vi "AlliGator Display Accumulated Dataset.vi"(8 "error in (no error)":errorcluster, 9 "Sum (F) or Average (T)":bool, 11 "AlliGator IV DVR in":refnum<data-value>) -> (0 "error out":errorcluster, 1 "Averaged?":bool, 2 "# Accumulated Datasets":i32, 3 "AlliGator IV DVR out":refnum<data-value>, 7 "Time-Series Folder":path)   [LabVIEW 2021, in "AlliGator Source Image.lvlib"]
doc: "Displays the Sum of all accumulated images or their mean, depending on the user-selected menu option."
uses:
  AlliGator Source Image.lvlib
  AlliGator Internal Variables v2.ctl
  <vilib>/vision/Image Controls.llb/IMAQ Image.ctl
  AlliGator Gate Image Set.ctl
  AlliGator FLI Dataset Type.ctl
  AlliGator Data Series Type.ctl
  AlliGator Dataset Channel.ctl
  AlliGator Gate Arithmetic.ctl
  AlliGator Displayed Image.ctl
  Image/Named ROI Description.ctl
  AlliGator Decay Metadata v3.ctl
  AlliGator Decay Background Subtraction Info.ctl
  AlliGator Baseline Subtraction Method.ctl
  Graphs/XY Graph/XY Graph Plot Shift Parameters.ctl
  Graphs/XY Graph/XY Graph Plot Shift Method.ctl
  AlliGator Decay Extrapolation Parameters.ctl
  Phasor/Calibration Phasor (m, phi).ctl
  Phasor/Phasor Reference Series.ctl
  Phasor/Phasor Calibration Map v2.ctl
  Phasor/Phasor (g, s).ctl
  AlliGator Raw Phasor Plot Data v4.ctl
  Phasor/Phasor Standard Deviation Options.ctl
  AlliGator Phasor Multi-Harmonic Data.ctl
  Phasor/Phasor Harmonic Data.ctl
  AlliGator Decay Fit Options & Parameters v2.ctl
  Fits/IRF(X)PSED/Decay Fit Options v2.ctl
  Fits/Decay Convolution/Decay Model.ctl
  Fits/Residual Type.ctl
  Fits/IRF(X)PSED/Fit Weights Type.ctl
  Fits/Non-linear Fitting Method v2.ctl
  Fits/Fit Calculation Method.ctl
  Fits/Non-linear Fitting Algorithm.ctl
  AlliGator Decay Fit Parameter Constraints 2.ctl
  Fits/IRF(X)PSED/Decay Fit Parameters In List.ctl
  Fits/IRF(X)PSED/MLE Baseline Offset Type.ctl
  AlliGator Decay Preprocessing Parameters.ctl
  Fits/IRF(X)PSED/Decay Fit Parameters & Derived Quantities List.ctl
  AlliGator Parameter Maps Data.ctl
  AlliGator Variables List.ctl
  Variant/Variant to Data/Variant to I32.vi
  Variant/Variant to Data/Variant to U16.vi
  <vilib>/vision/NI_Vision_Development_Module.lvlib
  Variant/Variant to Data/Variant to Data.lvlib
  AlliGator Globals, Variables & Constants.lvlib
  Utilities/Utilities.lvlib
  Phasor/Phasor.lvlib
  Image/Image.lvlib
  AlliGator Internal Variables.lvlib
  AlliGator Files.lvlib
  AlliGator Phasor Graph.lvlib
  AlliGator Decay Preprocessing.lvlib
  Graphs/XY Graph/XY Graph Add-Ons.lvlib
  AlliGator Phasor Plot.lvlib
  Fits/Fits.lvlib
  AlliGator Decay Fit.lvlib
  AlliGator Decay Fit Parameter Map.lvlib
  AlliGator Settings.lvlib
  AlliGator Dual-Channel Datasets.lvlib
panel:
  # "see the AlliGator License on the block diagram (Ctrl+E or Window:Show Block Diagram)"
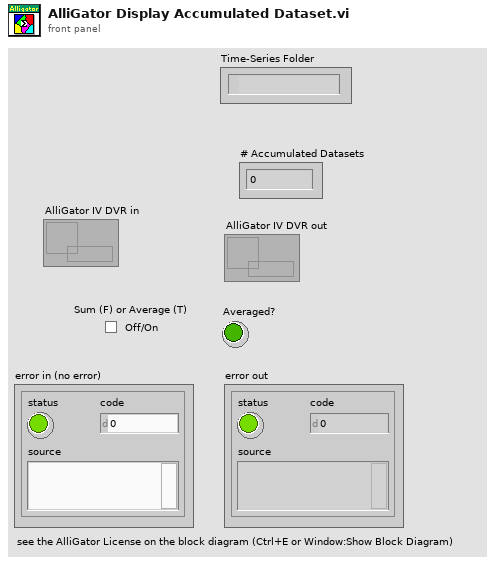
[diagram p1: front panel]
types:
  T1 = typedef "AlliGator Globals, Variables & Constants.lvlib/AlliGator Variables List.ctl" = enum16{"---- GUI ----", "GUI:Initialization Status", "GUI:State Indicators Refnum", "GUI:Original AlliGator Menu Items", "GUI:Current Action Loop State", "GUI:Script in progress", "GUI:Playback", "GUI:Loop Playback", "GUI:Search ROI Used", "GUI:Search ROI", "Decay Graph Max Legend Size", "Intensity Graph Max Legend Size", "Decay Statistics Graph Max Legend Size", "Phasor Graph Max Legend Size", "Phasor Ratio Graph Max Legend Size", "Lifetime Graph Max Legend Size", "---- Files ----", "Files:Export Dataset Frames as Individual Files", "Files:Show Batch Export Help Balloons", "Files:Frames in Dataset", "Files:ptu File Frame Start Indices", "Files:Current Frame in Dataset", "Files:Current Frame Timestamp", "Files:Dataset Loaded", "Files:Dataset Metadata", "Files:Dataset Channel", "Files:Dataset Data Description", "Files:Background Dataset Metadata", "Files:Background Dataset Channel", "Files:Background Dataset Data Description", "Files:Background File Subtraction", "Files:Background File Path", "Files:Background File Pile-up Correction", "Files:Background File Pixel Well Capacity", "Files:Background File Scaling Factor", "Files:Current Dataset Load Settings", "Files:Dataset Path", "------ Python Plugins ------", "Python Plugins:Information", "Python Plugins:Python Session", "Python Plugins:Valid Python Session?", "---- Source Image ----", "Source Image:ROIs", "Source Image:Current ROI", "Source Image:ROI Event Refnum", "X_Source Image Display Range", "X_Source Image Palette Information", "Source Image:Palette List", "Source Image:Scale", "Source Image:ROI Overlay Color", "Source Image:ICCD-specific Information", "Source Image:Overlay to Erase", "Source Image:Is Displayed Image Accumulated", "---- Image Profile Window ----", "Image Profile:Overlay ROI in Source Image", "Image Profile Window Event Refnum", "Image Profile:IntensityType", "Image Profile:Intensity Average Type", "Image Profile:Intensity-weighted SDV", "Image Profile:Box Profile Type", "Image Profile Window Open", "Image Profile:Plotted Fit Parameter", "X_Type of Displayed Image", "X_Time Gate Slider", "White Light Image Modified", "Mask Image Modified", "Macrotime Gate Separation", "------ Phasor Graph -------", "Phasor Graph:Show Line", "---- Phasor Plot ---", "Phasor Plot Parameters Changed", "FLI Dataset Modified since last Phasor Plot Calculation", "Phasor Harmonics Data", "Selected Phasor Harmonics", "Phasor Harmonic Manager Event Refnum", "Phasor Plot ROIs", "Current Phasor Plot ROI", "Phasor Plot ROI Event Refnum", "Phasor Plot Image Reference Points", "Phasor Plot Computed", "Phasor Plot Palette Information", "Phasor Plot Palette List", "Phasor Ratio Palette Information", "Phasor Ratio Palette List", "Phasor Image Scale", "Phasor Plot Image Overlay to Erase", "Phasor Plot Image Elements to Update", "Current Phasor Plot Calculation Parameters", "Current Phasor Calibration Options", "Reset Cumulated Phasor Plot", "Phasor Ratio Reference 1", "Phasor Ratio Lifetime Reference 1", "Phasor Ratio Reference 1 Frequency", "Phasor Ratio Reference 2", "Phasor Ratio Lifetime Reference 2", "Phasor Ratio Reference 2 Frequency", "---- Decay Analysis ----", "Number of Selected Decays to Fit", "LS Fit Results", "LAR Fit Results", "BS Fit Results", "Last Decay Max - Min", "Best Fit Parameters", "Best Fit Parameter Names", "Actual Size X", "Actual Size Y", "Binning X", "Binning Y", "Actual # Gates", "Dataset Number", "Gates to...", "Gates Skipped", "Gates to keep", "Gate Step", "Gate Separation", "Reversed Gates", "Pile-up Correction", "Pixel Well Capacity", "Background Subtracted", "Background Subtraction Method", "Background Definition Range", "Background File (deprecated)", "Number of Dataset Accumulated", "Array of Accumulated Dataset Paths", "Do Averaged Datasets", "Destination File Path", "Process Plot Target", "Use 1/D as Phasor Frequency", "---- Decay Fit Parameter Map -----", "Decay Fit Parameter Map Palette Information", "Decay Fit Parameter Map Palette List", "Local Decay Graph Window Event Refnum", "------- Local Decay Window ---------", "Use normalized IRF for convolution", "----- Miscellaneous ----", "Skippable Dialog Windows Status"}
  T2 = typedef "AlliGator Internal Variables.lvlib/AlliGator Internal Variables v2.ctl" = cluster{"Displayed Image":T3, "White Light Image":T3, "Mask Image":T3, "ROI Mask Image":T3, "Current Dataset Images 1":T4, "Background Dataset Images 1":T4, "Current Dataset Images 2":T4, "Background Dataset Images 2":T4, "Current Dataset Arithmetic Images":T4, "Accumulated Dataset Images 1":T4, "Accumulated Dataset Images 2":T4, "Accumulated Dataset Arithmetic Images":T4, "Phasor Plot Image":T3, "Decay Fit Parameter Map Image":T3, "Single Data Point Path":path, "White Light Image Path":path, "Mask Image Path":path, "Time-Series Folder":path, "[Time-Series Paths]":path[], "Current Dataset":i32, "Single Dataset Type":T5, "Current Folder":string, "AlliGator Data Series Type":T6, "# Datasets":i32, "Dual-Channel Dataset":bool, "Selected Channel Name":string, "Dataset Channel":T7, "Channel Arithmetic":T8, "Dual-Channel Background Dataset":bool, "Background Channel":T7, "Dual-Channel Accumulated Dataset":bool, "Start Time":dbl, "[Time-Series Timestamps]":dbl[], "[Intensity Corrections]":dbl[], "Time Series Script":bool, "Type of Displayed Image":T9, "Gate Image Slide":u16, "# Gates":i32, "ROIs":T10[], "ROI Decay":cluster{"t Array":dbl[], "I Array":dbl[]}, "Valid Decay":bool, "Decay  Metadata":T12, "Reference Decay Plot Name":string, "Reference Decay":cluster{"t Array":dbl[], "I Array":dbl[]}, "Decay Shift Plot":cluster{"Time Stamps":dbl[], "Decay Shifts":dbl[]}, "[Decays Max Values]":sgl[], "[Decays Min Values]":sgl[], "Calibration Phasor":T18, "Calibration Phasor Series":T19, "Phasor Calibration Map":T20, "Calibration Map MD5 Digest":string, "Last Raw Phasor":T21, "Last Calibrated Phasor":T21, "Last Calibrated Phasor SDV":T21, "Phasor Graph:Phasor Plot":cluster{"g Array":dbl[], "s Array":dbl[]}, "Phasor Graph:Phasor SDV Plot":cluster{"g Array":dbl[], "s Array":dbl[]}, "[Phasor Graph:Raw Phasor Plots]":T22[], "Phasor Plot locked to Ref 1":i32, "[Phasor Plot(s) locked to Ref 1]":i32[], "[Phasor Plot(s) locked to Ref 2]":i32[], "[Pixel Phasors]":T21[], "[[Sum Image]]":dbl[][], "[[CSG Phasors]]":csg[][], "[[Valid Pixel?]]":bool[][], "I/m/phi Dataset":cluster{"I/m/phi Dataset?":bool, "Base Frequency":dbl[unit], "Harmonic Orders":u8[]}, "Multi Phasor Plot Data":T24, "Decay Fit Options & Parameters":T26, "Fit Options: Decay Preprocessing Parameters":T37, "Fit Options: Reference Decay":cluster{"t Array":dbl[], "I Array":dbl[]}, "Is Full Image Parameters Map":bool, "Is Single-Pixels Parameters Map":bool, "NLSF Parameters Map X Resolution":i32, "NLSF Parameters Map Y Resolution":i32, "[Single Decay Fit Parameters]":dbl[], "Fit Model":T28, "[[Multiple Decays Fit Parameters]]":dbl[][], "[[Multiple Decays Fit Parameter SDVs]]":dbl[][], "[[IRFs]]":dbl[][], "IRF Array Time Axis":dbl[], "Decay Array Time Axis":dbl[], "[Decay Fit Parameter Names]":T38[], "[[Phasor Ratios]]":dbl[][], "[[Average Lifetimes]]":dbl[][], "Amplitude Weighted Average Lifetime":bool, "[Decay Sum]":dbl[], "Parameter Maps":T39[], "[[User-defined Quantities]]":dbl[][], "User-defined Quantity":string}
  T3 = typedef "IMAQ Image.ctl" = refnum<image>
  T4 = typedef "AlliGator Internal Variables.lvlib/AlliGator Gate Image Set.ctl" = cluster{"SGL Image Max":T3, "SGL Image Sum":T3, "SGL Gate Images":T3[], "SGL Image Min":T3}
  T5 = typedef "AlliGator Files.lvlib/AlliGator FLI Dataset Type.ctl" = enum16{"HDF5 FLI Dataset", "Gate Image Folder", ".sdt FLI Dataset (Becker & Hickl)", ".ptu FLI Dataset (PicoQuant)", "SS1 FLI Dataset", "SS2 FLI Dataset", "I/m/phi Dataset", ".bin FLI Dataset (PicoQuant Binned)", ".bin FLI Dataset (Piccolo Binned)"}
  T6 = typedef "AlliGator Files.lvlib/AlliGator Data Series Type.ctl" = enum16{"Not a Supported Series", "Gate Images Folder Series", "SwissSPAD 2 Dataset Series", "B&H FLI Dataset Series", "PicoQuant PTU FLI Dataset Series", "PicoQuant BIN FLI Dataset Series", "Piccolo hist BIN FLI Dataset Series", "HDF5 FLI Dataset Series"}
  T7 = typedef "AlliGator Dual-Channel Datasets.lvlib/AlliGator Dataset Channel.ctl" = enum16{"G2", "INT"}
  T8 = typedef "AlliGator Settings.lvlib/AlliGator Gate Arithmetic.ctl" = enum16{"None", "INT-G2", "G2/INT*<INT>", "(1 - G2/INT)*<INT>"}
  T9 = typedef "AlliGator Source Image.lvlib/AlliGator Displayed Image.ctl" = enum16{"Single Gate", "Sum of All Gates", "Max of All Gates", "Min of All Gates", "-", "White Ligth Image", "Mask Image"}
  T10 = typedef "Image.lvlib/Named ROI Description.ctl" = cluster{"ROI Descriptor":T11, "ROI Name":string, "Overlay Color":u32}
  T11 = typedef "ROI Descriptor" = cluster{"Global Rectangle":i32[], "Contours":cluster{"ID":enum32{"External", "Internal"}, "Type":u32, "Coordinates":i32[]}[]}
  T12 = typedef "AlliGator Phasor Graph.lvlib/AlliGator Decay Metadata v3.ctl" = cluster{"ROI Descriptor":T11, "ROI Center":cluster{"X":i32, "Y":i32}, "Decay Background Subtraction Info":T13, "Decay Reverted":bool, "Decay Smoothened":bool, "Decay Straightened":bool, "Fitted Tau (Decay Straightening)":dbl, "Decay Shift Parameters":T15, "Decay Shifted":bool, "Decay Extrapolated":bool, "Decay Extrapolation Parameters":T17, "Decay Normalized":bool, "Fold Decay":bool, "# Folds":u32}
  T13 = typedef "AlliGator Decay Analysis.lvlib/AlliGator Decay Preprocessing.lvlib/AlliGator Decay Background Subtraction Info.ctl" = cluster{"Laser Period":dbl[unit], "Gate Duration":dbl[unit], "Baseline Subtraction Method":T14, "Background Definition Range":cluster{"Min Gate":dbl[unit], "Max Gate":dbl[unit]}, "Total Intensity w/o Bkgd Subtraction":dbl, "Bkgd-subtracted Intensity (exp)":dbl, "# Data Points":i32, "Background/Gate":dbl, "Fitted Lifetime":dbl[unit], "Bkgd-subtracted Intensity (theo)":dbl}
  T14 = typedef "AlliGator Decay Analysis.lvlib/AlliGator Decay Preprocessing.lvlib/AlliGator Baseline Subtraction Method.ctl" = enum16{"Mean", "Min", "Square Gated Single-Exponential", "File", "Constant"}
  T15 = typedef "XY Graph Add-Ons.lvlib/XY Graph Plot Shift Parameters.ctl" = cluster{"Type":T16, "Shift":dbl[unit], "Threshold":dbl, "Rotate":bool}
  T16 = typedef "XY Graph Add-Ons.lvlib/XY Graph Plot Shift Method.ctl" = enum16{"Default", "CFD", "Threshold", "Cross-Correlation"}
  T17 = typedef "AlliGator Decay Analysis.lvlib/AlliGator Decay Preprocessing.lvlib/AlliGator Decay Extrapolation Parameters.ctl" = cluster{"Additional Points":u32, "Head Fraction":dbl, "Fitted Tau":dbl, "Use Periodicity":bool, "Use Cursors":bool, "Tail Fraction":dbl}
  T18 = typedef "Phasor.lvlib/Calibration Phasor (m, phi).ctl" = cluster{"m":dbl, "phi":dbl, "Phasor Frequency":dbl[unit], "Reference Lifetime":dbl[unit]}
  T19 = typedef "Phasor.lvlib/Phasor Reference Series.ctl" = cluster{"m Array":dbl[], "phi Array":dbl[], "Phasor Frequency":dbl[unit], "Calibration Lifetime":dbl[unit]}
  T20 = typedef "Phasor.lvlib/Phasor Calibration Map v2.ctl" = cluster{"Phasor Frequency":dbl[unit], "Calibration Lifetime":dbl[unit], "ROI Centers":cluster{"X":i32, "Y":i32}[], "ROI Descriptors":T11[], "Map Resolution X":i32, "Map Resolution Y":i32, "z Array":cdb[]}
  T21 = typedef "Phasor.lvlib/Phasor (g, s).ctl" = cluster{"g":dbl, "s":dbl}
  T22 = typedef "AlliGator Phasor Graph.lvlib/AlliGator Raw Phasor Plot Data v4.ctl" = cluster{"Phasor Plot Name":string, "Raw Phasor Plot":T21[], "Phasor Frequency":dbl[unit], "[Decay Metadata]":T12[], "Raw Phasor Plot SDV":T21[], "Phasor SDV Options":T23, "[Calibration Phasor]":T18[]}
  T23 = typedef "Phasor.lvlib/Phasor Standard Deviation Options.ctl" = cluster{"Compute Estimated SDV":bool, "# Replicas":u32, "Use Estimated Average Phasor":bool}
  T24 = typedef "AlliGator Phasor Plot.lvlib/AlliGator Phasor Multi-Harmonic Data.ctl" = cluster{"Base Frequency":dbl[unit], "# Harmonics":u8, "Harmonic Orders":u8[], "Phasor Plot Settings Checksum":u64, "Phasor Harmonic Data Array":T25[]}
  T25 = typedef "Phasor.lvlib/Phasor Harmonic Data.ctl" = cluster{"Phasor Harmonic Name":string, "Phasor Plot Settings Checksum":u64, "Phasor Frequency":dbl[unit], "Base Frequency":dbl[unit], "Harmonic Order":u8, "Phasor Plot Parameters":string, "Phasor Array [[CSG]]":csg[][], "Dataset File Path":path}
  T26 = typedef "AlliGator Decay Fit Parameter Map.lvlib/AlliGator Decay Fit Options & Parameters v2.ctl" = cluster{"SYNC Period":dbl[unit], "Fit Options":T27, "Fit Parameter Constraints":T34[], "MLE Baseline Offset":dbl, "MLE Baseline Offset Type":T36}
  T27 = typedef "Fits.lvlib/Decay Fit Options v2.ctl" = cluster{"Show Fit Residuals":bool, "Fit Model":T28, "Residual Type":T29, "Max Decay Percentile":dbl, "Min Decay Percentile":dbl, "Show Full Decay":bool, "Weights":T30, "Fitting Method":T31, "Compute Parameter Uncertainties":bool, "Periodic Boundaries":bool, "Model Calculation":T32, "Period":dbl[unit], "Termination Criteria":cluster{"Max Iterations":i32, "Max Function Calls":i32, "Max Time":dbl[unit], "Function Tolerance":dbl, "Parameter Tolerance":dbl, "Gradient Tolerance":dbl, "Min Lambda":dbl, "Max Lambda":dbl, "Initial Tick Count":u32}, "Offset Resolution":dbl[unit], "Use Local IRF":bool, "Fitting Algorithm":T33}
  T28 = typedef "Fits.lvlib/Decay Model.ctl" = enum16{"1-Exponential", "2-Exponentials"}
  T29 = typedef "Fits.lvlib/Residual Type.ctl" = enum16{"Standard", "Normalized", "Reduced"}
  T30 = typedef "Fits.lvlib/Fit Weights Type.ctl" = enum16{"Unweighted", "1/Variance", "Best of All"}
  T31 = typedef "Fits.lvlib/Non-linear Fitting Method v2.ctl" = enum16{"Least Square", "Least Absolute Residual", "Bisquare", "MLE", "-", "Best of All"}
  T32 = typedef "Fits.lvlib/Fit Calculation Method.ctl" = enum16{"Simulation", "Convolution", "Integration"}
  T33 = typedef "Fits.lvlib/Non-linear Fitting Algorithm.ctl" = enum16{"Levenberg-Marquardt", "Trust-Region Dogleg"}
  T34 = typedef "AlliGator Decay Analysis.lvlib/AlliGator Decay Fit.lvlib/AlliGator Decay Fit Parameter Constraints 2.ctl" = cluster{"Fit Parameter":T35, "Min Value":dbl, "Max Value":dbl, "Global":bool, "Used":bool}
  T35 = typedef "Fits.lvlib/Decay Fit Parameters In List.ctl" = enum16{"Offset", "Baseline", "A_1", "tau_1", "A_2", "tau_2"}
  T36 = typedef "Fits.lvlib/MLE Baseline Offset Type.ctl" = enum32{"Absolute", "Percentage"}
  T37 = typedef "AlliGator Decay Analysis.lvlib/AlliGator Decay Preprocessing.lvlib/AlliGator Decay Preprocessing Parameters.ctl" = cluster{"Background Subtraction":bool, "Straighten Decay":bool, "Reverse Gates":bool, "1-Normalized Decay":bool, "Smoothen Decay":bool, "Smoothing Parameter":dbl, "Shift Decay":bool, "Decay Shift Parameters":T15, "Extrapolate Decay":bool, "Additional Points":u32, "Head Fraction":dbl, "Pixel-Normalize Decay":bool, "Use Periodicity":bool, "Use Cursors":bool, "Tail Fraction":dbl, "Use Decay Pre-Processing":bool, "Fold Decay":bool, "# Folds":u32, "[0-1]-Normalized Decay":bool}
  T38 = typedef "Fits.lvlib/Decay Fit Parameters & Derived Quantities List.ctl" = enum16{"Offset", "Baseline", "A_1", "tau_1", "A_2", "tau_2", "<tau>_a", "f1_a", "f2_a", "<tau>_i", "f1_i", "f2_i", "-", "R^2", "Chi^2"}
  T39 = typedef "AlliGator Parameter Maps Data.ctl" = cluster{"Map Set Name":string, "[Parameter Names]":string[], "[[Parameters]]":dbl[][], "[[Parameter SDVs]]":dbl[][], "Decay Array Time Axis":dbl[], "[[IRFs]]":dbl[][], "IRF Array Time Axis":dbl[]}
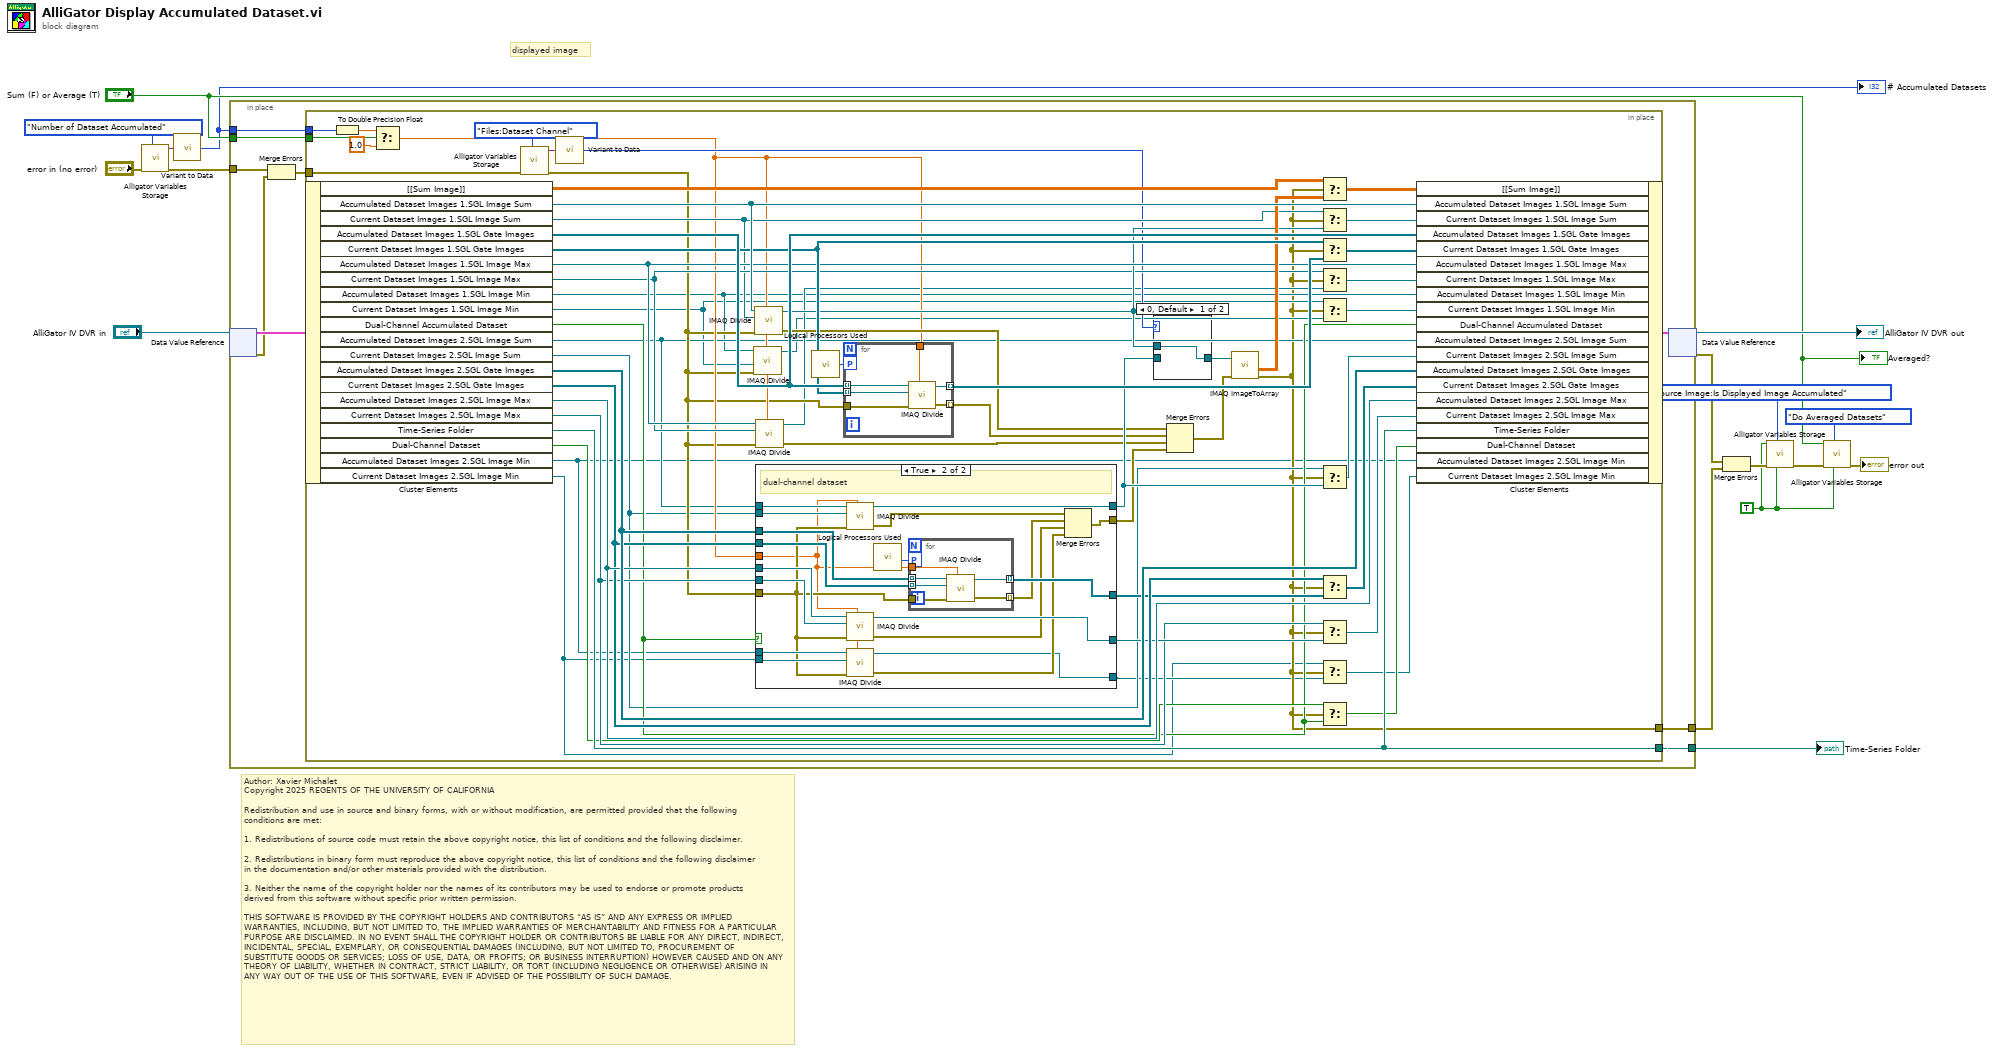
[diagram p0: block diagram]
diagram:
  w6 = TRUE ("Averaged?")
  # "Author: Xavier Michalet\nCopyright 2025 REGENTS OF THE UNIVERSITY OF CALIFORNIA\n\nRedistribution and use in source and binary forms, with or without modification, are permitted provided that the following conditions are met:\n\n1. Redistributions of source code must retain the above copyright notice, this list of conditions and the following disclaimer.\n\n2. Redistributions in binary form must reproduce the above copyright notice, this list of conditions and the following disclaimer in the documentation and/or other materials provided with the distribution.\n\n3. Neither the name of the copyright holder nor the names of its contributors may be used to endorse or promote products derived from this software without specific prior written permission.\n\nTHIS SOFTWARE IS PROVIDED BY THE COPYRIGHT HOLDERS AND CONTRIBUTORS “AS IS” AND ANY EXPRESS OR IMPLIED WARRANTIES, INCLUDING, BUT NOT LIMITED TO, THE IMPLIED WARRANTIES OF MERCHANTABILITY AND FITNESS FOR A PARTICULAR PURPOSE ARE DISCLAIMED. IN NO EVENT SHALL THE COPYRIGHT HOLDER OR CONTRIBUTORS BE LIABLE FOR ANY DIRECT, INDIRECT, INCIDENTAL, SPECIAL, EXEMPLARY, OR CONSEQUENTIAL DAMAGES (INCLUDING, BUT NOT LIMITED TO, PROCUREMENT OF SUBSTITUTE GOODS OR SERVICES; LOSS OF USE, DATA, OR PROFITS; OR BUSINESS INTERRUPTION) HOWEVER CAUSED AND ON ANY THEORY OF LIABILITY, WHETHER IN CONTRACT, STRICT LIABILITY, OR TORT (INCLUDING NEGLIGENCE OR OTHERWISE) ARISING IN ANY WAY OUT OF THE USE OF THIS SOFTWARE, EVEN IF ADVISED OF THE POSSIBILITY OF SUCH DAMAGE."
  # "displayed image"
  n1 = call "Alligator Variables Storage.vi"("AlliGator Variable"=AlliGator_Variables_List."Number of Dataset Accumulated" ("Alligator Variable"), "Error In"="error in (no error)") -> ("Error Out"=w2:errorcluster, "Data out"=w12:variant)  [unwired: 7 in, 1 out]
  n2 = call-poly "Variant to Data.vi"("Variant"=w12) -> ("Value"=w3:i32)  [unwired: 8 in]
  "# Accumulated Datasets" <- w3
  n3 = in-place {
    in-place-border: "Sum (F) or Average (T)" -> [w25]
    in-place-border: w3 -> [w24]
    in-place-border: [w22] -> w10
    in-place-border: w2 -> [w21]
    in-place-border: [w18] -> w1
    n4 = in-place-dvr #1("AlliGator IV DVR in") -> (w26:T2, w20:errorcluster)
    n5 = Merge Errors(w21, w20) -> (w19:errorcluster)
    n6 = in-place {
      in-place-border: w25 -> [w50]
      in-place-border: w24 -> [w69]
      in-place-border: [w31] -> w22
      in-place-border: w19 -> [w43]
      in-place-border: [w59] -> w18
      n7 = in-place-cluster #2(w26) -> ("[[Sum Image]]"=w73:dbl[][], "Accumulated Dataset Images 1.SGL Image Sum"=w83:T3, "Current Dataset Images 1.SGL Image Sum"=w47:T3, "Accumulated Dataset Images 1.SGL Gate Images"=w82:T3[], "Current Dataset Images 1.SGL Gate Images"=w79:T3[], "Accumulated Dataset Images 1.SGL Image Max"=w74:T3, "Current Dataset Images 1.SGL Image Max"=w70:T3, "Accumulated Dataset Images 1.SGL Image Min"=w36:T3, "Current Dataset Images 1.SGL Image Min"=w35:T3, "Dual-Channel Accumulated Dataset"=w56:bool, "Accumulated Dataset Images 2.SGL Image Sum"=w37:T3, "Current Dataset Images 2.SGL Image Sum"=w32:T3, "Accumulated Dataset Images 2.SGL Gate Images"=w68:T3[], "Current Dataset Images 2.SGL Gate Images"=w63:T3[], "Accumulated Dataset Images 2.SGL Image Max"=w67:T3, "Current Dataset Images 2.SGL Image Max"=w60:T3, "Time-Series Folder"=w59:path, "Dual-Channel Dataset"=w57:bool, "Accumulated Dataset Images 2.SGL Image Min"=w29:T3, "Current Dataset Images 2.SGL Image Min"=w28:T3)
      n8 = To Double Precision Float(number=w69) -> (double precision float=w49:dbl)
      n9 = Select(t=w49, s=w50, f=1.0) -> (s? t:f=w40:dbl)
      n10 = call "Alligator Variables Storage.vi"("AlliGator Variable"=AlliGator_Variables_List."Files:Dataset Channel" ("Alligator Variable"), "Error In"=w43) -> ("Error Out"=w39:errorcluster, "Data out"=w45:variant)  [unwired: 7 in, 1 out]
      n11 = call-poly "Variant to Data.vi"("Variant"=w45) -> ("U16 Value"=w44:u16)  [unwired: 8 in]
      n12 = call "IMAQ Divide"("Image Src A"=w36, "Constant"=w40, "Image Src B"=w35, "error in (no error)"=w39) -> ("Image Dst Out"=w34:T3)  [unwired: 3 in, 1 out]
      n13 = call "IMAQ Divide"("Image Src A"=w83, "Constant"=w40, "Image Dst"=w47, "error in (no error)"=w39) -> ("Image Dst Out"=w72:T3, "error out"=w52:errorcluster)  [unwired: 3 in]
      n14 = call "IMAQ Divide"("Image Src A"=w74, "Constant"=w40, "Image Dst"=w70, "error in (no error)"=w39) -> ("Image Dst Out"=w38:T3, "error out"=w53:errorcluster)  [unwired: 3 in]
      n15 = case shown="True" w56 {
        tunnel: w39 -> [_ w93]
        tunnel: w40 -> [_ w92]
        tunnel: w37 -> [_ w109]
        tunnel: w32 -> [w89 w108]
        tunnel: w68 -> [_ w107]
        tunnel: w63 -> [w88 w106]
        tunnel: w67 -> [_ w105]
        tunnel: w60 -> [w87 w104]
        tunnel: [w89 w103] -> w58
        tunnel: [w88 w102] -> w62
        tunnel: [w87 w101] -> w61
        tunnel: [_ w100] -> w42
        tunnel: w28 -> [w86 w95]
        tunnel: [w86 w90] -> w30
        tunnel: w29 -> [_ w94]
        frame False {
          # "not a dual-channel dataset"
        }
        frame True {
          # "dual-channel dataset"
          n16 = call "IMAQ Divide"("Image Src A"=w109, "Constant"=w92, "Image Dst"=w108, "error in (no error)"=w93) -> ("Image Dst Out"=w103:T3, "error out"=w97:errorcluster)  [unwired: 3 in]
          n17 = call "IMAQ Divide"("Image Src A"=w105, "Constant"=w92, "Image Dst"=w104, "error in (no error)"=w93) -> ("Image Dst Out"=w101:T3, "error out"=w98:errorcluster)  [unwired: 3 in]
          n18 = call "IMAQ Divide"("Image Src A"=w94, "Constant"=w92, "Image Dst"=w95, "error in (no error)"=w93) -> ("Image Dst Out"=w90:T3, "error out"=w91:errorcluster)  [unwired: 3 in]
          n19 = call "Logical Processors Used.vi"() -> ("# Logical Processor Used"=w96:i32)  [unwired: 6 in]
          n20 = for {
            tunnel: w107 -> [w112] mode=indexing
            tunnel: w106 -> [w111] mode=indexing
            tunnel: [w114] -> w99 mode=indexing
            tunnel: w93 -> [w115]
            tunnel: [w113] -> w102 mode=indexing
            workers-P: w96 -> [_]
            tunnel: w92 -> [w110]
            n21 = call "IMAQ Divide"("Image Src A"=w112, "Constant"=w110, "Image Dst"=w111, "error in (no error)"=w115) -> ("Image Dst Out"=w113:T3, "error out"=w114:errorcluster)  [unwired: 3 in]
          }
          n22 = Merge Errors(w97, w99, w98, w91) -> (w100:errorcluster)
        }
      }
      n23 = call "Logical Processors Used.vi"() -> ("# Logical Processor Used"=w51:i32)  [unwired: 6 in]
      n24 = for {
        tunnel: w82 -> [w118] mode=indexing
        tunnel: w79 -> [w117] mode=indexing
        tunnel: [w120] -> w54 mode=indexing
        tunnel: w39 -> [w121]
        tunnel: [w119] -> w81 mode=indexing
        workers-P: w51 -> [_]
        tunnel: w40 -> [w116]
        n25 = call "IMAQ Divide"("Image Src A"=w118, "Constant"=w116, "Image Dst"=w117, "error in (no error)"=w121) -> ("Image Dst Out"=w119:T3, "error out"=w120:errorcluster)  [unwired: 3 in]
      }
      n26 = case shown="0, Default" w44 {
        tunnel: [w84 w85] -> w71
        tunnel: w58 -> [_ w85]
        tunnel: w72 -> [w84 _]
        frame 0, Default {
        }
        frame 1 {
        }
      }
      n27 = Merge Errors(w52, w54, w53, w42) -> (w41:errorcluster)
      n28 = call "IMAQ ImageToArray"("error in (no error)"=w41, "Image"=w71) -> ("Image Pixels (Float)"=w75:sgl[][], "error out"=w31:errorcluster)  [unwired: 2 in, 3 out]
      n29 = Select(t=w73, s=w31, f=w75) -> (s? t:f=w76:dbl[][])
      n30 = Select(t=w47, s=w31, f=w72) -> (s? t:f=w77:T3)
      n31 = Select(t=w79, s=w31, f=w81) -> (s? t:f=w80:T3[])
      n32 = Select(t=w70, s=w31, f=w38) -> (s? t:f=w78:T3)
      n33 = Select(t=w35, s=w31, f=w34) -> (s? t:f=w33:T3)
      n34 = Select(t=w32, s=w31, f=w58) -> (s? t:f=w66:T3)
      n35 = Select(t=w63, s=w31, f=w62) -> (s? t:f=w65:T3[])
      n36 = Select(t=w60, s=w31, f=w61) -> (s? t:f=w64:T3)
      n37 = Select(t=w28, s=w31, f=w30) -> (s? t:f=w27:T3)
      n38 = Select(t=w57, s=w31, f=w56) -> (s? t:f=w55:bool)
      n39 = in-place-cluster #2("[[Sum Image]]"=w76, "Accumulated Dataset Images 1.SGL Image Sum"=w83, "Current Dataset Images 1.SGL Image Sum"=w77, "Accumulated Dataset Images 1.SGL Gate Images"=w82, "Current Dataset Images 1.SGL Gate Images"=w80, "Accumulated Dataset Images 1.SGL Image Max"=w74, "Current Dataset Images 1.SGL Image Max"=w78, "Accumulated Dataset Images 1.SGL Image Min"=w36, "Current Dataset Images 1.SGL Image Min"=w33, "Dual-Channel Accumulated Dataset"=w56, "Accumulated Dataset Images 2.SGL Image Sum"=w37, "Current Dataset Images 2.SGL Image Sum"=w66, "Accumulated Dataset Images 2.SGL Gate Images"=w68, "Current Dataset Images 2.SGL Gate Images"=w65, "Accumulated Dataset Images 2.SGL Image Max"=w67, "Current Dataset Images 2.SGL Image Max"=w64, "Time-Series Folder"=w59, "Dual-Channel Dataset"=w55, "Accumulated Dataset Images 2.SGL Image Min"=w29, "Current Dataset Images 2.SGL Image Min"=w27) -> (w23:T2)
    }
    n40 = in-place-dvr #1(w23) -> (→"AlliGator IV DVR out":refnum<data-value>, w15:errorcluster)
  }
  "Time-Series Folder" <- w1
  n41 = Merge Errors(w15, w10) -> (w9:errorcluster)
  n42 = call "Alligator Variables Storage.vi"("Get(F)/Set"=w6, "AlliGator Variable"=AlliGator_Variables_List."Source Image:Is Displayed Image Accumulated" ("Alligator Variable"), "Error In"=w9, "Data in"=w6) -> ("Error Out"=w7:errorcluster)  [unwired: 5 in, 2 out]
  n43 = call "Alligator Variables Storage.vi"("Get(F)/Set"=w6, "AlliGator Variable"=AlliGator_Variables_List."Do Averaged Datasets" ("Alligator Variable"), "Error In"=w7, "Data in"="Sum (F) or Average (T)") -> ("Error Out"=→"error out":errorcluster)  [unwired: 5 in, 2 out]
  "Averaged?" <- "Sum (F) or Average (T)"
